vi "pickSurroundingPlatforms_multiPlatform.vi"(8 "Max number of platforms to \npick":i32=2, 9 "previousChoices":i32[][](array[numeric]), 10 "Goal \nplatform":i32, 11 "Start platform":i32) -> (3 "platform choices":i32[](array[numeric]))   [LabVIEW 2017]
panel:
  out "distance of \nchoices":dbl[](array[numeric])
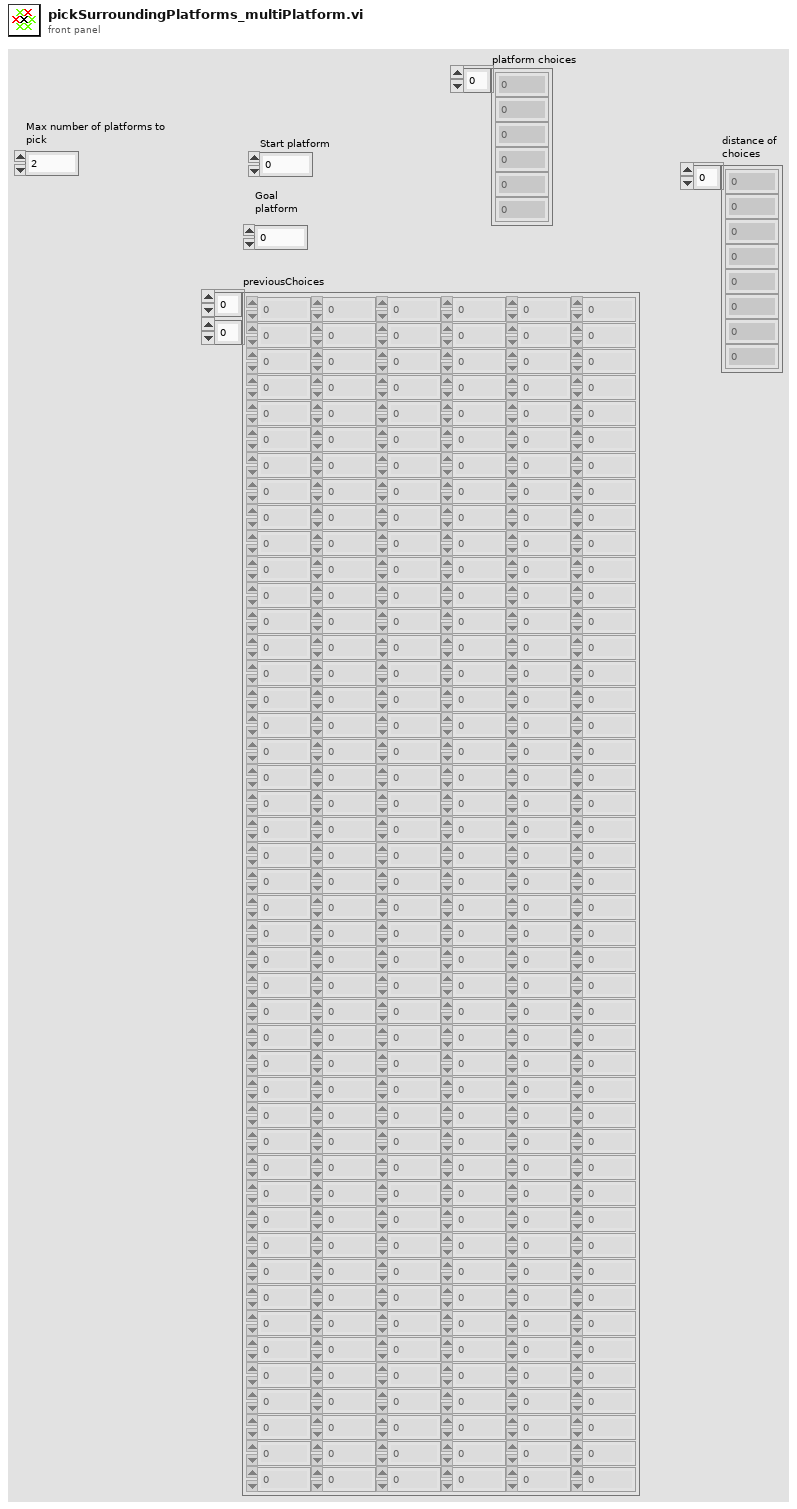
[diagram p1: front panel]
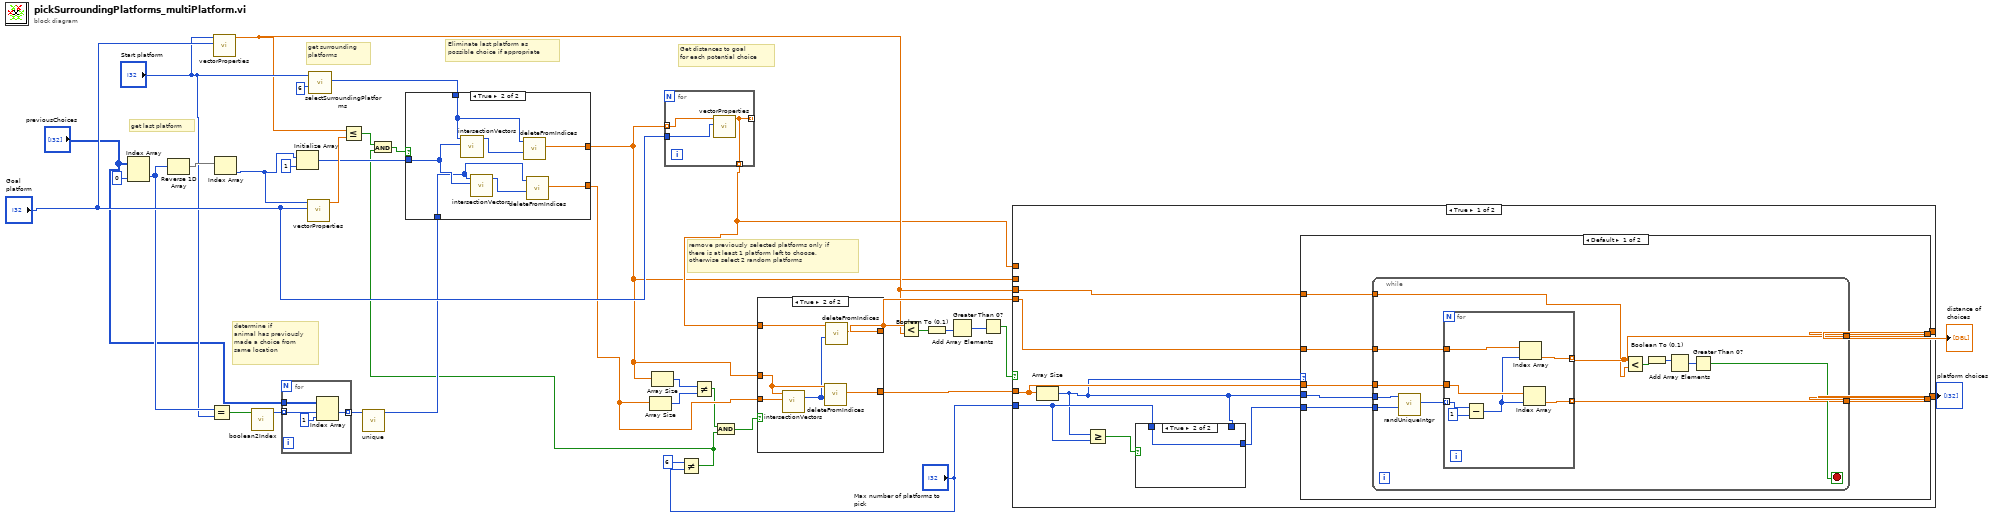
[diagram p0: block diagram]
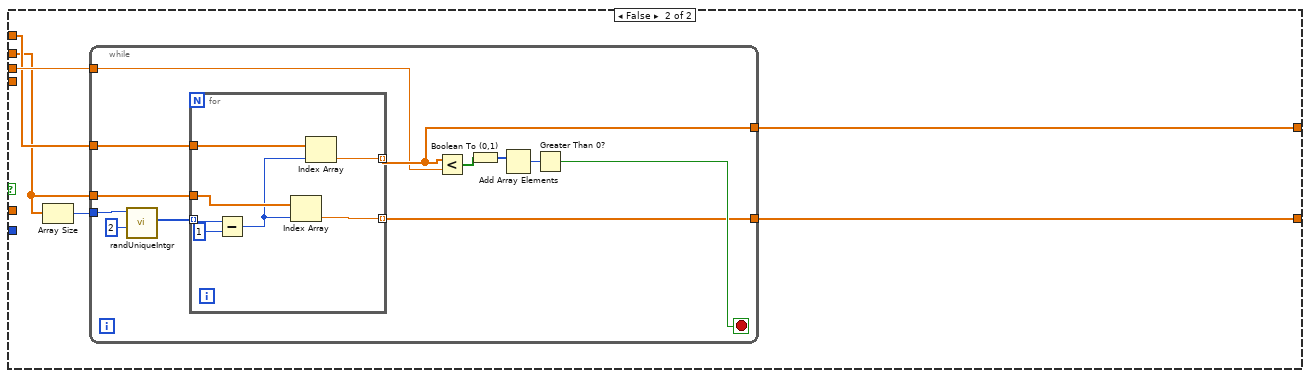
[diagram p4: hidden frame]
diagram:
  # "remove previously selected platforms only if \nthere is at least 1 platform left to choose,\notherwise select 2 random platforms"
  # "determine if \nanimal has previously \nmade a choice from \nsame location"
  # "Get distances to goal\nfor each potential choice"
  # "Eliminate last platform as \npossible choice if appropriate"
  # "get last platform"
  # "get surrounding\nplatforms"
  n1 = Index Array(array="previousChoices", index (col)=0 ("disabled index (col)")) -> (element=w26:i32[])  [unwired: 1 in]
  n2 = Reverse 1D Array(array=w26) -> (reversed array=w35:i32[])
  n3 = Equal?(x=w26, y="Start platform") -> (x = y?=w30:bool[])
  n4 = call "vectorProperties.vi"("Goal \nplatform"="Goal \nplatform", "Start \nplatform"="Start platform") -> ("vector length"=w13:dbl)  [unwired: 8 in, 1 out]
  n5 = Index Array(array=w35) -> (element=w33:i32)  [unwired: 1 in]
  n6 = call "boolean2Index.vi"("boolean"=w30) -> ("index"=w29:i32[])  [unwired: 10 in]
  n7 = for {
    tunnel: w29 -> [w40] mode=indexing
    tunnel: "previousChoices" -> [w41]
    tunnel: [w38] -> w23 mode=indexing
    n8 = Index Array(array=w41, index (row)=w40, index (col)=1) -> (element=w38:i32)
  }
  n9 = Initialize Array(w33, 1 ("dimension size")) -> (w32:i32[])
  n10 = call "vectorProperties.vi"("Goal \nplatform"="Goal \nplatform", "Start \nplatform"=w33) -> ("vector length"=w34:dbl)  [unwired: 8 in, 1 out]
  n11 = call "selectSurroundingPlatforms.vi"("Number of surrounding\nplatforms to raise"=6 ("Number of surrounding\nplatforms to raise"), "Start platform"="Start platform") -> ("Platforms \nto raise"=w22:i32[])  [unwired: 9 in]
  n12 = Less Or Equal?(x=w13, y=w34) -> (x <= y?=w2:bool)
  n13 = call "unique.vi"("Array"=w23) -> ("Array 2"=w21:i32[])  [unwired: 10 in]
  n14 = Not Equal?(x=6, y="Max number of platforms to \npick") -> (x != y?=w1:bool)
  n15 = And(x=w2, y=w1) -> (x .and. y?=w3:bool)
  n16 = case shown="True" w3 {
    tunnel: w22 -> [w43 w49]
    tunnel: w32 -> [_ w47]
    tunnel: [w43 w48] -> w11
    tunnel: w21 -> [w42 w45]
    tunnel: [w42 w44] -> w19
    frame False {
    }
    frame True {
      n17 = call "intersectionVectors.vi"("vector2"=w47, "vector1"=w49) -> ("vector1 indices"=w50:i32[])  [unwired: 8 in, 1 out]
      n18 = call "intersectionVectors.vi"("vector2"=w47, "vector1"=w45) -> ("vector1 indices"=w46:i32[])  [unwired: 8 in, 1 out]
      n19 = call "deleteFromIndices.vi"("indices to delete"=w50, "vector"=w49) -> ("vector restricted"=w48:dbl[])  [unwired: 9 in]
      n20 = call "deleteFromIndices.vi"("indices to delete"=w46, "vector"=w45) -> ("vector restricted"=w44:dbl[])  [unwired: 9 in]
    }
  }
  n21 = Array Size(array=w19) -> (size(s)=w27:i32)
  n22 = Array Size(array=w11) -> (size(s)=w28:i32)
  n23 = for {
    tunnel: w11 -> [w53] mode=indexing
    tunnel: "Goal \nplatform" -> [w52]
    tunnel: [w51] -> _ mode=indexing
    tunnel: [w51] -> w12 mode=indexing
    n24 = call "vectorProperties.vi"("Goal \nplatform"=w52, "Start \nplatform"=w53) -> ("vector length"=w51:dbl)  [unwired: 8 in, 1 out]
  }
  n25 = Not Equal?(x=w28, y=w27) -> (x != y?=w5:bool)
  n26 = And(x=w5, y=w1) -> (x .and. y?=w4:bool)
  n27 = case shown="True" w4 {
    tunnel: [w55 w61] -> w20
    tunnel: w11 -> [w55 w60]
    tunnel: w19 -> [_ w59]
    tunnel: w12 -> [w54 w58]
    tunnel: [w54 w56] -> w14
    frame False {
    }
    frame True {
      n28 = call "intersectionVectors.vi"("vector2"=w59, "vector1"=w60) -> ("vector1 indices"=w57:i32[])  [unwired: 8 in, 1 out]
      n29 = call "deleteFromIndices.vi"("indices to delete"=w57, "vector"=w60) -> ("vector restricted"=w61:dbl[])  [unwired: 9 in]
      n30 = call "deleteFromIndices.vi"("indices to delete"=w57, "vector"=w58) -> ("vector restricted"=w56:dbl[])  [unwired: 9 in]
    }
  }
  n31 = Less?(x=w14, y=w13) -> (x < y?=w18:bool[])
  n32 = Boolean To (0,1)(Boolean=w18) -> (0, 1=w16:i16[])
  n33 = Add Array Elements(numeric array=w16) -> (sum=w17:i16)
  n34 = Greater Than 0?(x=w17) -> (x > 0?=w15:bool)
  n35 = case shown="True" w15 {
    tunnel: w20 -> [w70 _]
    tunnel: w14 -> [w69 _]
    tunnel: w13 -> [w68 w105]
    tunnel: [w67 w104] -> w10
    tunnel: w12 -> [_ w103]
    tunnel: w11 -> [_ w102]
    tunnel: [w66 w101] -> w9
    tunnel: "Max number of platforms to \npick" -> [w64 _]
    frame True {
      n36 = Array Size(array=w70) -> (size(s)=w62:i32)
      n37 = Greater Or Equal?(x=w62, y=w64) -> (x >= y?=w65:bool)
      n38 = case shown="True" w65 {
        tunnel: w64 -> [_ w72]
        tunnel: [w71 w72] -> w63
        tunnel: w62 -> [w71 _]
        frame False {
        }
        frame True {
        }
      }
      n39 = case shown="Default" w62 {
        tunnel: w62 -> [w79 _]
        tunnel: w70 -> [w78 w99]
        tunnel: w69 -> [w77 w100]
        tunnel: w68 -> [w76 _]
        tunnel: [w75 w99] -> w67
        tunnel: [w74 w100] -> w66
        tunnel: w63 -> [w73 _]
        frame Default {
          n40 = while {
            tunnel: w79 -> [w91]
            tunnel: w78 -> [w89]
            tunnel: w77 -> [w88]
            tunnel: w76 -> [w81]
            tunnel: [w83] -> w75
            tunnel: [w82] -> w74
            tunnel: w73 -> [w80]
            stop <- w84 stop-if-true
            n41 = call "randUniqueIntgr.vi"("max rand number"=w91, "Number of Outputs"=w80) -> ("output"=w90:u32[])  [unwired: 8 in]
            n42 = for {
              tunnel: w90 -> [w94] mode=indexing
              tunnel: w89 -> [w98]
              tunnel: w88 -> [w97]
              tunnel: [w96] -> w82 mode=indexing
              tunnel: [w95] -> w83 mode=indexing
              n43 = Subtract(x=w94, y=u32 1) -> (x-y=w93:u32)
              n44 = Index Array(array=w97, index=w93) -> (element=w96:dbl)
              n45 = Index Array(array=w98, index=w93) -> (element=w95:dbl)
            }
            n46 = Less?(x=w82, y=w81) -> (x < y?=w85:bool[])
            n47 = Boolean To (0,1)(Boolean=w85) -> (0, 1=w87:i16[])
            n48 = Add Array Elements(numeric array=w87) -> (sum=w86:i16)
            n49 = Greater Than 0?(x=w86) -> (x > 0?=w84:bool)
          }
        }
        frame 1 {
        }
      }
    }
    frame False {
      n50 = Array Size(array=w102) -> (size(s)=w106:i32)
      n51 = while {
        tunnel: w106 -> [w118]
        tunnel: w102 -> [w115]
        tunnel: w103 -> [w114]
        tunnel: w105 -> [w107]
        tunnel: [w109] -> w104
        tunnel: [w108] -> w101
        stop <- w110 stop-if-true
        n52 = call "randUniqueIntgr.vi"("max rand number"=w118, "Number of Outputs"=2) -> ("output"=w116:u32[])  [unwired: 8 in]
        n53 = for {
          tunnel: w116 -> [w121] mode=indexing
          tunnel: w115 -> [w125]
          tunnel: w114 -> [w124]
          tunnel: [w123] -> w108 mode=indexing
          tunnel: [w122] -> w109 mode=indexing
          n54 = Subtract(x=w121, y=u32 1) -> (x-y=w120:u32)
          n55 = Index Array(array=w125, index=w120) -> (element=w122:dbl)
          n56 = Index Array(array=w124, index=w120) -> (element=w123:dbl)
        }
        n57 = Less?(x=w108, y=w107) -> (x < y?=w111:bool[])
        n58 = Boolean To (0,1)(Boolean=w111) -> (0, 1=w113:i16[])
        n59 = Add Array Elements(numeric array=w113) -> (sum=w112:i16)
        n60 = Greater Than 0?(x=w112) -> (x > 0?=w110:bool)
      }
    }
  }
  "platform choices" <- w10
  "distance of \nchoices" <- w9
